vi "InitCanon.vi"(8 "error in":errorcluster) -> (0 "error out":errorcluster)   [LabVIEW 2013]
uses:
  ROS/Code/SubVIs/BaxterSide.ctl
  ROS/Code/Console/Servers/ServerSubs/(nist) Arm Globals.vi
  NIST2/Prim/Fwd Kenimatics - array.vi
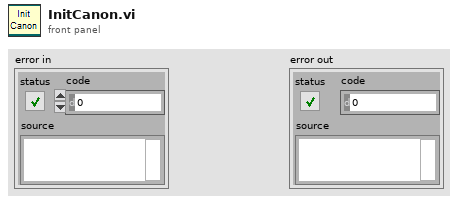
[diagram p1: front panel]
types:
  T1 = typedef "BaxterSide.ctl" = enum16{"left", "right"}
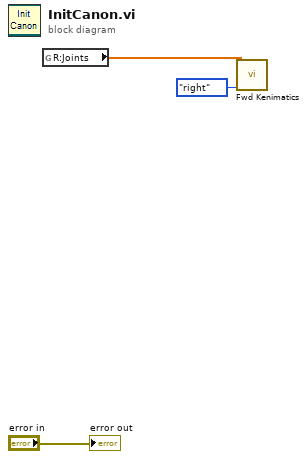
[diagram p0: block diagram]
diagram:
  n1 = global read "(nist) Arm Globals.vi" "R:Joints"() -> (w1:dbl[])
  n2 = call-poly "Fwd Kenimatics.vi"("Side"=BaxterSide."right", "Joints"=w1) -> ()  [unwired: 8 in, 2 out]
  "error out" <- "error in"
